vi "Callback - EventHappened.vi"(4 "Gauge":refnum<vi>, 5 "Event Data":cluster{"dValue":dbl}, 6 "Control Ref":refnum<k24>, 7 "Event Common Data":T1) -> ()   [LabVIEW 2023]
doc: "This callback VI runs whenever the DoubleValue property is set on the DataWatcher .NET object."
uses:
  c:/dev/_r/4/eng/lv-core/lvpostprocessingd/lv_mc_x86_64/dist_i386/examples/Connectivity/Dot NET/EventExample.dll
  EventExample.dll
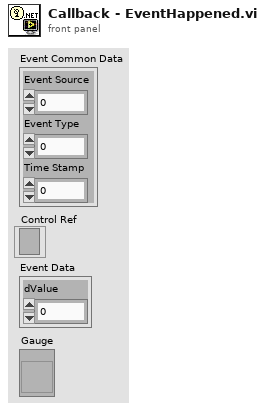
[diagram p1: front panel]
types:
  T1 = cluster{"Event Source":i32, "Event Type":u32, "Time Stamp":u32}
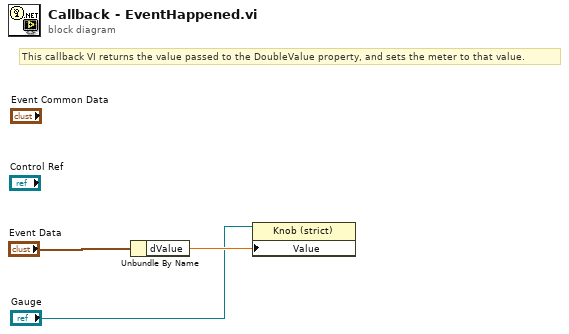
[diagram p0: block diagram]
diagram:
  # "This callback VI returns the value passed to the DoubleValue property, and sets the meter to that value."
  n1 = Unbundle By Name("Event Data") -> ("dValue"=w3:dbl)
  n2 = property class="Knob (strict)"(reference="Gauge", "Value"=w3) -> ()  [unwired: 1 in, 2 out]
